vi "Dashboard Main.vi"() -> ()   [LabVIEW 2018]
uses:
  <vilib>/Utility/miscctls.llb/LVRowAndColumnTypeDef.ctl
  <vilib>/event_ctls.llb/eventvkey.ctl
  <vilib>/Rock Robotics/Network Tables/NT Read Numeric Array.vi
  <vilib>/Rock Robotics/WPI/Dashboard/WPI_DashboardLogging Global.vi
panel:
  in  "Camera Settings Right":T1={"Frame Rate"=30, "Compression"=30, "Size"=1, "DB Camera Config"=FALSE} {"Frame Rate" scale=1.0..30.0; "Compression" scale=100.0..-1.0; "Size" items=["640x480", "320x240", "160x120"]}
  in  "Camera Name Right":string(combo)="No Camera Selection"
  out "Camera Perf":string
  in  "Camera Settings":T1={"Frame Rate"=30, "Compression"=30, "Size"=1, "DB Camera Config"=FALSE} {"Frame Rate" scale=1.0..30.0; "Compression" scale=100.0..-1.0; "Size" items=["640x480", "320x240", "160x120"]}
  in  "TCP":refnum<k5>
  in  "Rec Mode":enum32{"Stop", "Record", "Playback"}(radio)
  out "Robot IP":string
  out "Image Message":string="Timeout in Camera Communications"
  in  "Dashboard Tab":T2(tab)
  in  "Select Auto":string(combo)="Select Autonomous ..."
  out "NT Connection":bool
  out "MotorChart R":cluster{"Numeric":dbl, "Numeric":dbl}(graph)
  out "MotorChart L":cluster{"Numeric":dbl, "Numeric":dbl}(graph)
  out "MotorSliders R":cluster{"MotorSlide1":dbl, "MotorSlide2":dbl} {"MotorSlide2" scale=-1.0..1.0 scale format="%#_2e"; "MotorSlide1" scale=-1.0..1.0 scale format="%#_2e"}
  out "MotorSliders L":cluster{"MotorSlide1":dbl, "MotorSlide2":dbl} {"MotorSlide2" scale=-1.0..1.0 scale format="%#_2e"; "MotorSlide1" scale=-1.0..1.0 scale format="%#_2e"}
  out "Gyro":dbl(knob) scale=0.0..360.0
  out "JS1 Z":dbl(slide) scale=-1.0..1.0 scale format="%#_2e"
  out "JS1 Graph":cluster{"X":dbl, "Y":dbl}[](graph)
  out "JS1 Buttons":T3
  out "JS2 Z":dbl(slide) scale=-1.0..1.0 scale format="%#_2e"
  out "JS2 Graph":cluster{"X":dbl, "Y":dbl}[](graph)
  out "JS2 Buttons":T3
  out "Mode":T4(ring)=enum."Auto Disabled"
  out "Right Camera Perf":cluster{"Bandwidth (Mbps)":dbl, "FPS":dbl}
  out "X Position":sgl
  out "Y Position":sgl
  out "Camera Image Right":T5(plugin-control)
  in  "DB/String 9":string
  in  "DB/String 8":string
  in  "DB/String 7":string
  in  "DB/String 6":string
  in  "DB/String 5":string
  in  "DB/String 4":string
  in  "DB/String 3":string
  in  "DB/String 2":string
  in  "DB/String 1":string
  in  "DB/String 0":string
  in  "DB/Slider 0":dbl(slide) scale=0.0..5.0
  in  "DB/Slider 1":dbl(slide) scale=0.0..5.0
  in  "DB/Slider 2":dbl(slide) scale=0.0..5.0
  in  "DB/Slider 3":dbl(slide) scale=0.0..5.0
  out "DB/LED 3":bool
  out "DB/LED 2":bool
  out "DB/LED 1":bool
  out "DB/LED 0":bool
  in  "DB/Button 3":bool
  in  "DB/Button 2":bool
  in  "DB/Button 1":bool
  in  "DB/Button 0":bool caption="New Name"
  in  "Intake Speed":dbl=0.7 min=-1.0 max=1.0 step=0.1 format="%#_2f"
  in  "Shooter Speed":dbl=0.7 min=-1.0 max=1.0 step=0.1 format="%#_2f"
  in  "Autonomous Sequence":string="Auto 1"
  in  "Select Drive Type":dbl=1.0
  in  "Drive Number":i8=2
  in  "Test Slider":dbl(slide) scale=0.0..100.0 scale format="%#_3g"
  in  "On/Off":bool caption="Solenoid"
  in  "Test Name":u16(ring) items=["Select the test to run..."]
  in  "Test Tree":string(tree)
  in  "Motor":cluster{"Value":dbl, "Enable":bool} {"Value" scale=-1.0..1.0 scale format="%#_3g"}
  out "Progress":T6 {"Test Progress" scale=0.0..100.0}
  in  "Rev/Fwd":cluster{"Forward":bool, "Reverse":bool}
  in  "Test Ring":u16(ring) items=["Monochrome", "Color"]
  out "Cmd Status":string
  in  "Execute Command":bool
  in  "Command Params":string[][](table)
  in  "Command Selection":i32(listbox)
  in  "CheckList":i32(listbox)
  out "Tree":string(tree)
  out "Camera Image":T5(plugin-control)
  out "Background":bool
  in  "Camera Name":string(combo)="No Camera Selection"
  # "HW"
  # "HW"
  # "Joysticks"
  # "Drive Motors"
  # "Front"
  # "Right"
  # "Left"
  # "Back"
  # "This tab is a great place for autonomous settings and robot-specific values.\nPlace controls and indicators inside this tab and match name to\nDashboard Variables on robot. You can also delete this comment."
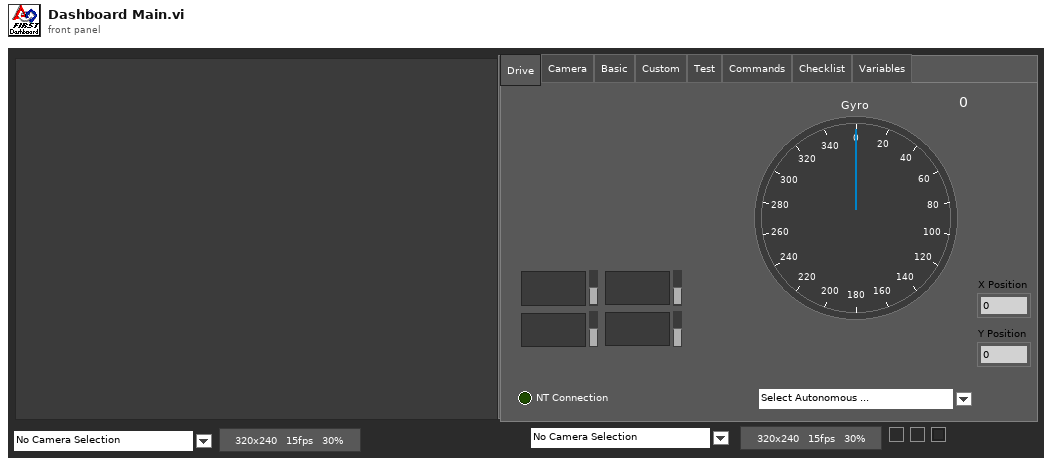
[diagram p1: front panel]
types:
  T1 = cluster{"Frame Rate":i32, "Compression":i32, "Size":u16, "DB Camera Config":bool}
  T2 = enum32{"Drive", "Camera", "Basic", "Custom", "Test", "Commands", "Checklist", "Variables"}
  T3 = cluster{bool, bool, bool, bool, bool, bool, bool, bool, bool, bool, bool, bool}
  T4 = enum8{"Tele-Op Disabled", "Tele-Op Enabled", "Auto Disabled", "Auto Enabled", "Test Disabled", "Test Enabled", "Disconnected", "No Code", "E-Stop"}
  T5 = typedef "IMAQ Image.ctl" = refnum<image>
  T6 = cluster{"Test Progress":u8, "Test Progress Text":string}
  T7 = cluster{"Save Path":path, "Interval (s)":dbl, "Keep":i32}
  T8 = typedef "Image Type" = u32
  T9 = cluster{"IDs":cluster{"RPC field ID":u16, "Unique ID":u16}, "String":string}
  T10 = cluster{"Camera Image":refnum<vi>, "Dashboard Tab":refnum<vi>, "Background":refnum<vi>, "Rec Mode":refnum<vi>, "Test Slider":refnum<vi>, "On/Off ":refnum<vi>, "Test Ring":refnum<vi>, "Rev/Fwd":refnum<vi>, "Test Name":refnum<vi>, "Motor":refnum<vi>, "Progress":refnum<vi>, "CheckList":refnum<vi>, "Tree":refnum<vi>, "Test Tree":refnum<vi>, "Command Params":refnum<vi>, "Command Selection":refnum<vi>, "Execute Command":refnum<vi>, "Cmd Status":refnum<vi>, "Camera Settings":refnum<vi>, "Camera Name":refnum<vi>, "Camera Perf":refnum<vi>, "Camera Settings Right":refnum<vi>, "Camera Name Right":refnum<vi>, "Camera Image Right":refnum<vi>}
  T11 = cluster{"Global Rectangle":i32[], "Contours":cluster{"Contour Type":u32, "ROI Type":u32, "Points":i32[]}[]}
  T12 = cluster{"Camera Name Right":string, string, "Saved DB Images Info":cluster{"Save Path":path, "Interval (s)":dbl, "Keep":i32}}
  T13 = cluster{"Error Strings":string, "Disable Counts":cluster{u16, u16}, "Rail Faults":cluster{u16, u16, u16}, "Robot IP":string, "DB Mode":u8, "Event Info":cluster{"Name":string, "Type":u8, "Number":u16, "Replay":u8}}
  T14 = cluster{"Storage":cluster{"Disk Free":u64, "RAM Block":u32, "RAM free":u32}, "CPU Utilization":cluster{"CPU % ISR":sgl, "CPU % Time Crit":sgl, "CPU % Timed Str":sgl, "CPU % High":sgl, "CPU % Above":sgl, "CPU % Normal":sgl, "CPU % Low":sgl}, "CAN":cluster{"% Bus Utilization":sgl, "Bus Off Cnt":u32, "TX_FIFO Full Cnt":u32, "Receive Error Cnt":u8, "Transmit Error Cnt":u8}, "HID":cluster{"HID Outputs":u32, "Rumble Low":u16, "Rumble High":u16}[]}
  T15 = cluster{"Status bits":cluster{"Test Mode":bool, "Autonomous":bool, "Enabled":bool, "Code Start":bool, "Brownout":bool, "Reserved 2":bool, "Reserved 3":bool, "E-Stop":bool}, "Code Trace":cluster{"Disabled":bool, "TeleOp":bool, "Auto":bool, "Test":bool}, "Controller Type":enum16{"unknown", "cRIO", "roboRio"}, "Code?":enum16{"unknown", "noCode", "code"}, "Battery V":dbl}
  T16 = cluster{"Control Bits":cluster{"TestMode":bool, "Autonomous":bool, "Enabled":bool, "FMS Present":bool, bool, bool, bool, "E-Stop":bool}, "Team Station ":u8, "Countdown":sgl, "Joystick Values":cluster{"Axes":dbl[], "Buttons":bool[], "POVs":i16[]}[]}
  T17 = cluster{"Axes":dbl[], "Buttons":bool[], "POVs":i16[]}[]
  T18 = cluster{"Axes":dbl[], "Buttons":bool[], "POVs":i16[]}
  T19 = cluster{"Buttons[0]":bool, "Buttons[1]":bool, "Buttons[2]":bool, "Buttons[3]":bool, "Buttons[4]":bool, "Buttons[5]":bool, "Buttons[6]":bool, "Buttons[7]":bool, "Buttons[8]":bool, "Buttons[9]":bool, "Buttons[10]":bool, "Buttons[11]":bool}
  T20 = cluster{"Camera Name":string, string, "Saved DB Images Info":cluster{"Save Path":path, "Interval (s)":dbl, "Keep":i32}}
  T21 = cluster{"Position":cluster{"x":sgl, "y":sgl}, "Angle":sgl, "Scale":sgl, "Score":sgl, "Bounding Box":cluster{"x":sgl, "y":sgl}[]}[]
  T22 = cluster{"Position":cluster{"x":sgl, "y":sgl}, "Angle":sgl, "Scale":sgl, "Score":sgl, "Bounding Box":cluster{"x":sgl, "y":sgl}[]}
  T23 = cluster{"Operation":enum16{"Update", "Clear"}, "Color Box":u32}[]
  T24 = typedef "eventvkey.ctl" = enum16{"ASCII", "Enter", "Return", "Shift", "Ctrl", "Alt", "Cmd", "Opt", "Caps", "NumLock", "Clear", "Break", "Up", "Down", "Left", "Right", "Insert", "Delete", "Home", "End", "PageUp", "PageDown", "Escape", "Help", "Pause", "ScrollLock", "F1", "F2", "F3", "F4", "F5", "F6", "F7", "F8", "F9", "F10", "F11", "F12", "F13", "F14", "F15", "F16", "F17", "F18", "F19", "F20", "F21", "F22", "F23", "F24", "Play", "VolumeUp", "VolumeDown", "Mute", "Two Byte Char"}
  T25 = cluster{"Image Size":bool, "Image Type":bool, "Pixel Value":bool, "ROI Information":bool, "Zoom Factor":bool}
  T26 = cluster{"Operation":enum16{"Update", "Clear"}, "Color Box":u32}
  T27 = typedef "LVRowAndColumnTypeDef.ctl" = cluster{"Row":i32, "Column":i32}
  T28 = cluster{"Shift":bool, "Ctrl":bool, "Alt":bool, "Cmd":bool, "Opt":bool}
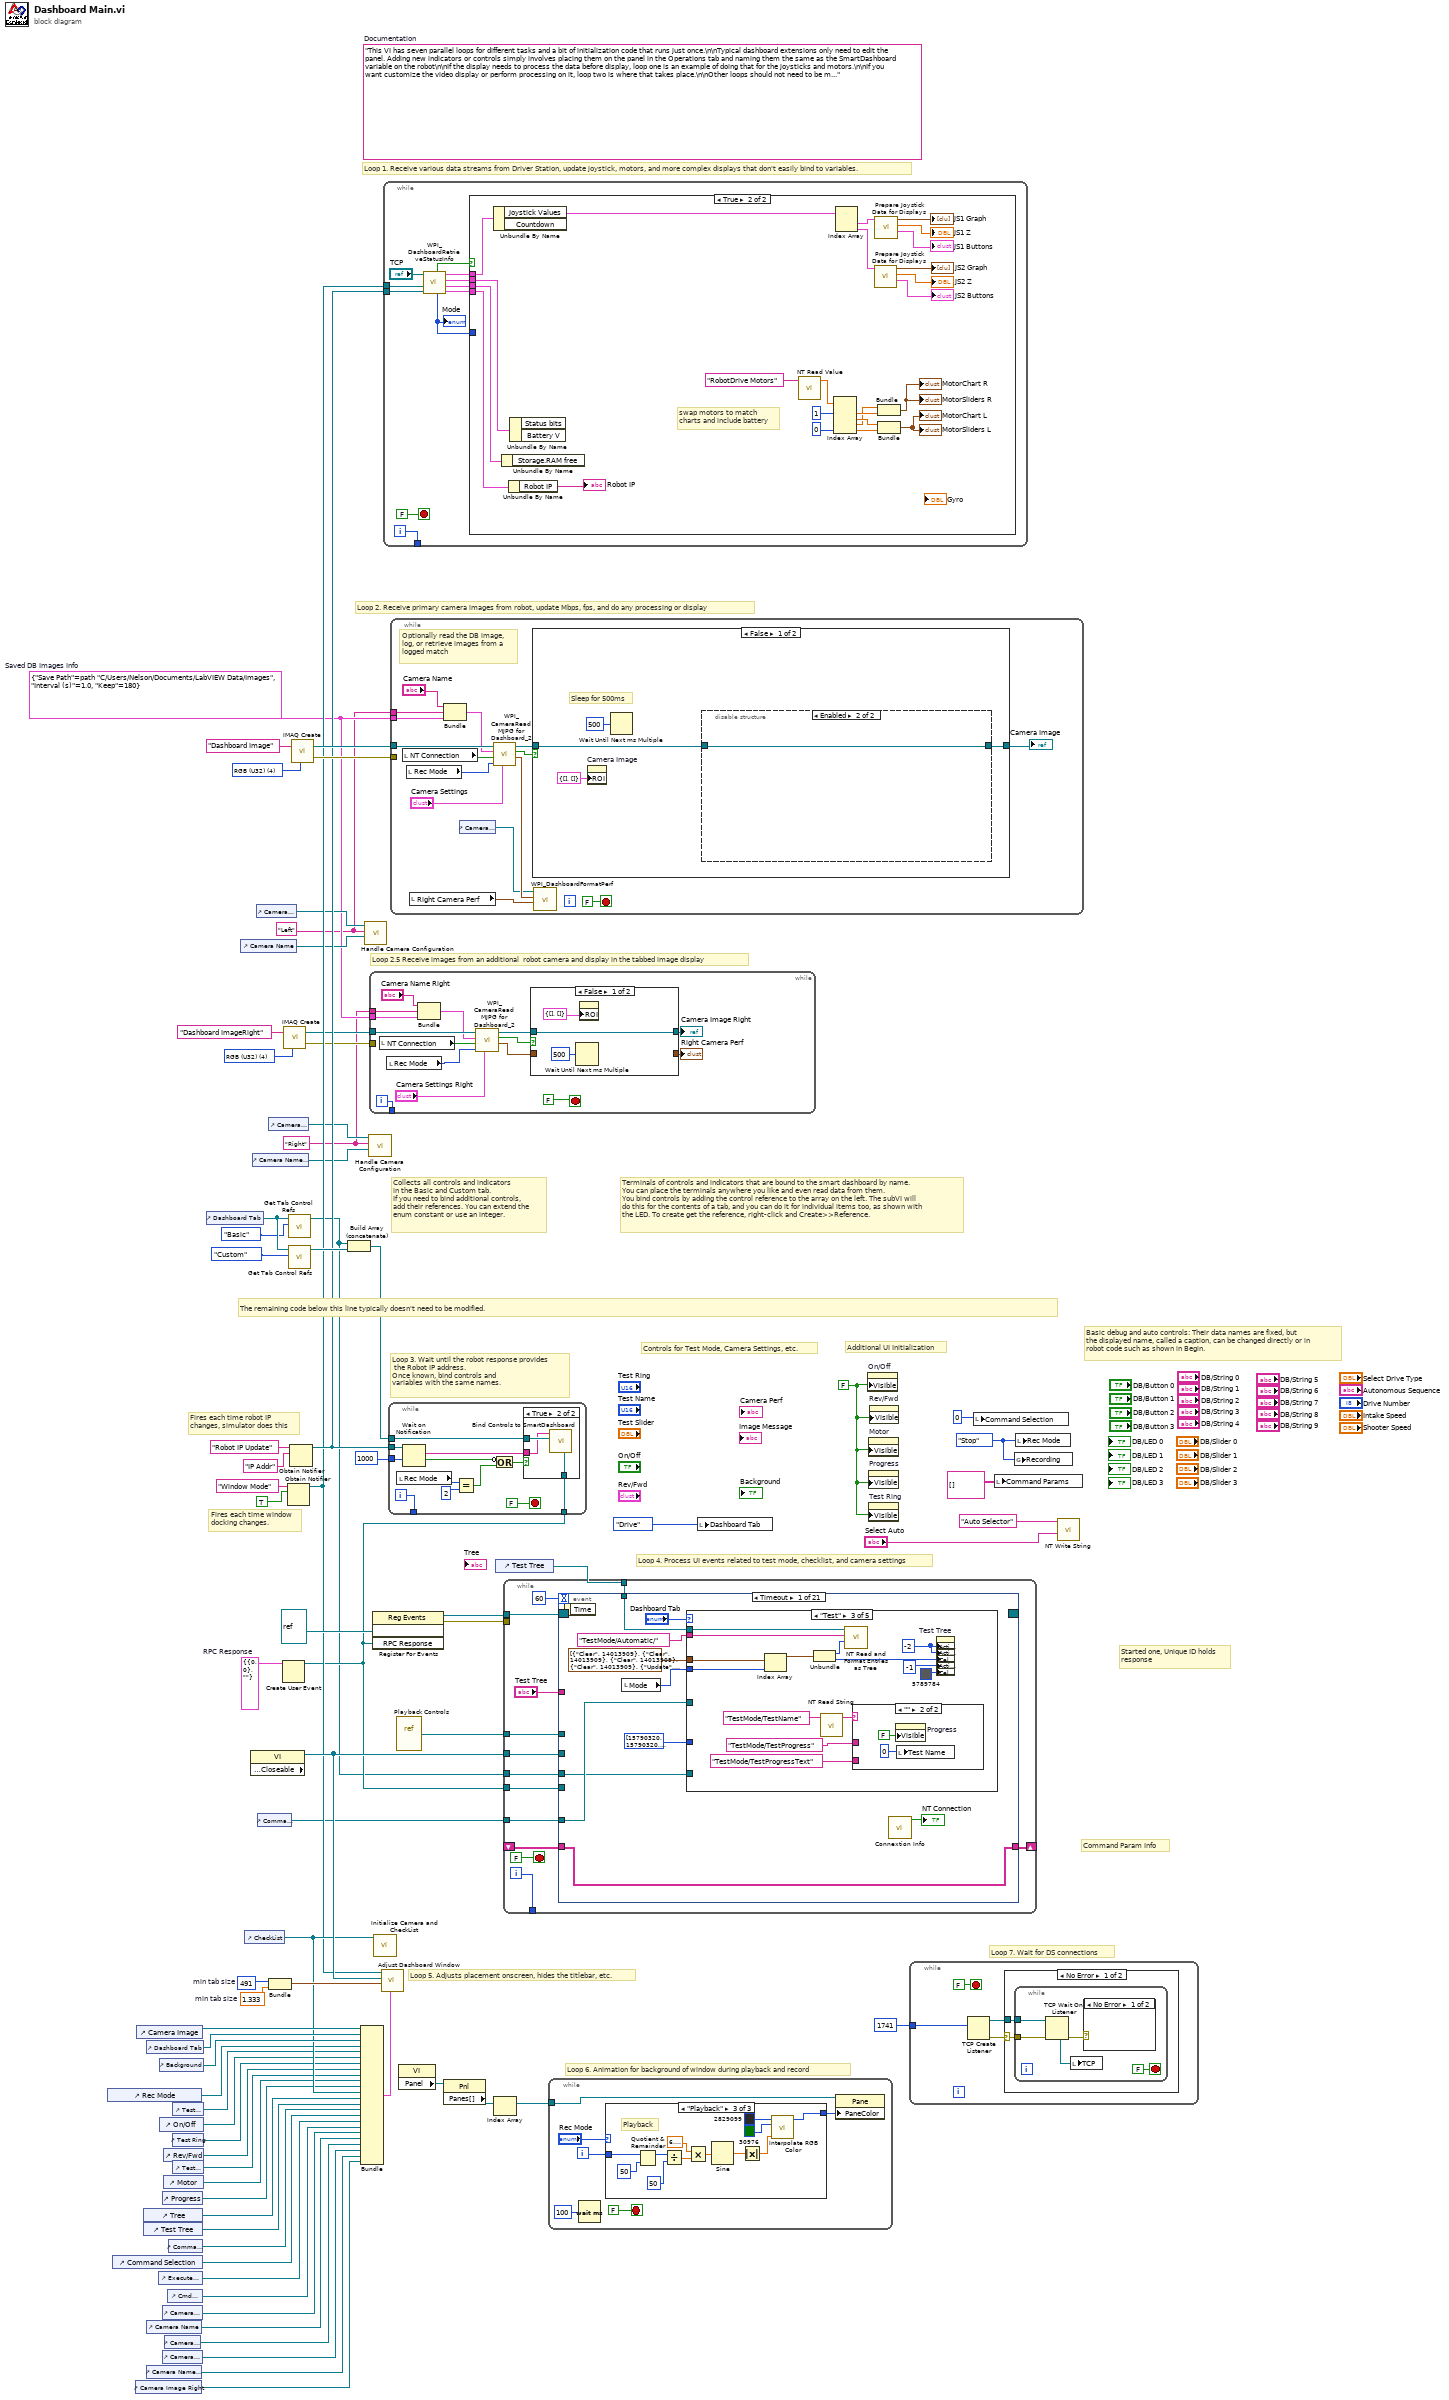
[diagram p0: block diagram]
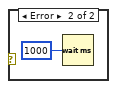
[diagram p3: hidden frame]
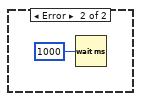
[diagram p4: hidden frame]
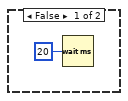
[diagram p5: hidden frame]
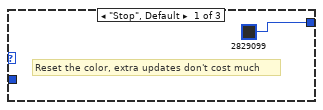
[diagram p6: hidden frame]
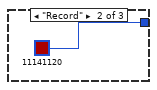
[diagram p7: hidden frame]
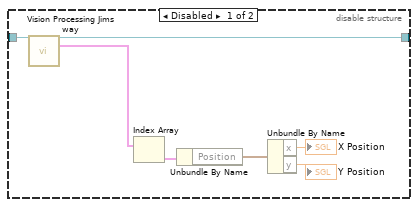
[diagram p9: hidden frame]
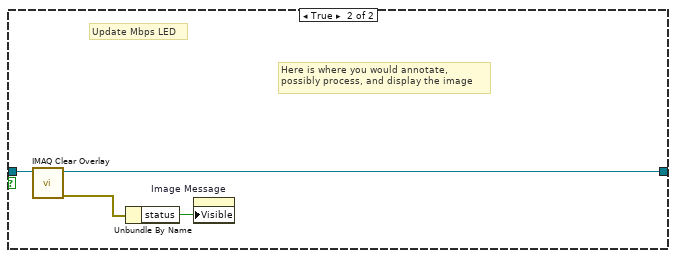
[diagram p10: hidden frame]
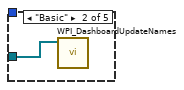
[diagram p12: hidden frame]
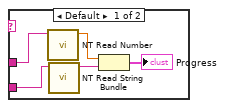
[diagram p13: hidden frame]
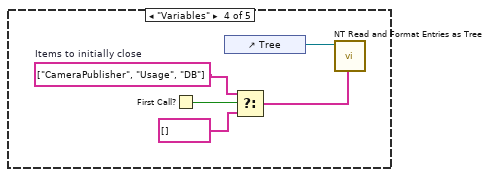
[diagram p14: hidden frame]
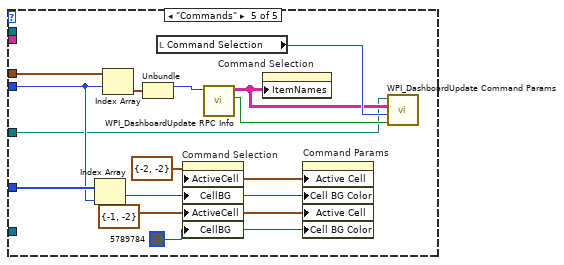
[diagram p15: hidden frame]
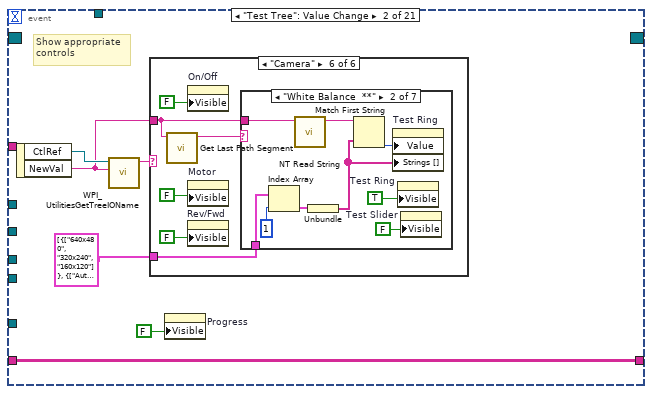
[diagram p16: hidden frame]
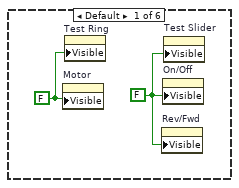
[diagram p17: hidden frame]
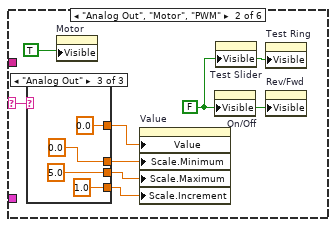
[diagram p18: hidden frame]
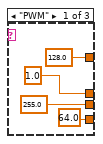
[diagram p19: hidden frame]
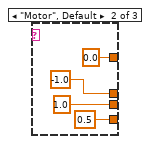
[diagram p20: hidden frame]
diagram:
  w3 = T7 {"Save Path"=path "C:/Users/Nelson/Documents/LabVIEW Data/Images", "Interval (s)"=1.0, "Keep"=180}  # Saved DB Images Info
  w2 = "Right"
  w1 = "Left"
  w13 = T8 4 items=["Grayscale (U8)", "Grayscale (I16)", "Grayscale (SGL)", "Complex (CSG)", "RGB (U32)", "HSL (U32)", "RGB (U64)"] ("Image Type")
  w29 = T9 {"IDs"={"RPC field ID"=0, "Unique ID"=0}, "String"=""}  # RPC Response
  w52 = 491  # min tab size
  w51 = 1.333  # min tab size
  w59 = enum32{"Stop", "Record", "Playback"}."Stop" ("Rec Mode")
  w36 = FALSE ("Visible")
  (unwired) "This VI has seven parallel loops for different tasks and a bit of initialization code that runs just once.\n\nTypical dashboard extensions only need to edit the panel. Adding new indicators or controls simply involves placing them on the panel in the Operations tab and naming them the same as the SmartDashboard variable on the robot\n\nIf the display needs to process the data before display, loop one is an example of doing that for the joysticks and motors.\n\nIf you want customize the video display or perform processing on it, loop two is where that takes place.\n\nOther loops should not need to be modified. They are pretty standard, and document the task they perform."  # Documentation
  w76 = T8 4 items=["Grayscale (U8)", "Grayscale (I16)", "Grayscale (SGL)", "Complex (CSG)", "RGB (U32)", "HSL (U32)", "RGB (U64)"] ("Image Type")
  # "Loop 2.5 Receive images from an additional  robot camera and display in the tabbed image display"
  # "Command Param Info"
  # "Started one, Unique ID holds\nresponse"
  # "Loop 7. Wait for DS connections"
  # "Basic debug and auto controls: Their data names are fixed, but\nthe displayed name, called a caption, can be changed directly or in\nrobot code such as shown in Begin."
  # "Controls for Test Mode, Camera Settings, etc."
  # "Additional UI Initialization"
  # "Loop 6. Animation for background of window during playback and record"
  # "Fires each time robot IP\nchanges, simulator does this"
  # "Fires each time window\ndocking changes."
  # "Collects all controls and indicators\nin the Basic and Custom tab.\nIf you need to bind additional controls,\nadd their references. You can extend the\nenum constant or use an integer."
  # "The remaining code below this line typically doesn't need to be modified."
  # "Loop 4. Process UI events related to test mode, checklist, and camera settings"
  # "Terminals of controls and indicators that are bound to the smart dashboard by name.\nYou can place the terminals anywhere you like and even read data from them.\nYou bind controls by adding the control reference to the array on the left. The subVI will\ndo this for the contents of a tab, and you can do it for individual items too, as shown with\nthe LED. To create get the reference, right-click and Create>>Reference."
  # "Loop 3. Wait until the robot response provides\n the Robot IP address.\nOnce known, bind controls and\nvariables with the same names."
  # "Loop 5. Adjusts placement onscreen, hides the titlebar, etc."
  # "Loop 1. Receive various data streams from Driver Station, update joystick, motors, and more complex displays that don't easily bind to variables."
  # "Loop 2. Receive primary camera images from robot, update Mbps, fps, and do any processing or display"
  n1 = control-ref of="Rec Mode"() -> (w42:refnum<vi>)
  n2 = control-ref of="Command Selection"() -> (w28:refnum<vi>)
  n3 = control-ref of="Camera Image Right"() -> (w6:refnum<vi>)
  n4 = control-ref of="Camera Image"() -> (w54:refnum<vi>)
  n5 = control-ref of="Tree"() -> (w46:refnum<vi>)
  n6 = control-ref of="Test Tree"() -> (w45:refnum<vi>)
  n7 = control-ref of="Dashboard Tab"() -> (w53:refnum<vi>)
  n8 = control-ref of="Camera Name"() -> (w19:refnum<vi>)
  n9 = control-ref of="Camera Name Right"() -> (w7:refnum<vi>)
  n10 = control-ref of="Execute Command"() -> (w30:refnum<vi>)
  n11 = control-ref of="Background"() -> (w49:refnum<vi>)
  n12 = control-ref of="On/Off"() -> (w40:refnum<vi>)
  n13 = control-ref of="Progress"() -> (w37:refnum<vi>)
  n14 = control-ref of="Camera Settings"() -> (w20:refnum<vi>)
  n15 = control-ref of="Camera Settings Right"() -> (w8:refnum<vi>)
  n16 = control-ref of="Rev/Fwd"() -> (w38:refnum<vi>)
  n17 = control-ref of="Motor"() -> (w43:refnum<vi>)
  n18 = control-ref of="Camera Perf"() -> (w18:refnum<vi>)
  n19 = control-ref of="Cmd Status"() -> (w24:refnum<vi>)
  n20 = control-ref of="Command Params"() -> (w31:refnum<vi>)
  n21 = control-ref of="Test Slider"() -> (w41:refnum<vi>)
  n22 = control-ref of="Test Ring"() -> (w39:refnum<vi>)
  n23 = control-ref of="Test Name"() -> (w44:refnum<vi>)
  n24 = control-ref of="Dashboard Tab"() -> (w57:refnum<vi>)
  n25 = control-ref of="Camera Name"() -> (w21:refnum<vi>)
  n26 = control-ref of="CheckList"() -> (w47:refnum<vi>)
  n27 = property class="VI" props=["Front Panel.Closeable"]() -> (reference out=w58:refnum<vi>)  [unwired: 2 in, 2 out]
  n28 = control-ref of="Camera Name Right"() -> (w9:refnum<vi>)
  n29 = control-ref of="Camera Settings"() -> (w22:refnum<vi>)
  n30 = control-ref of="Command Params"() -> (w23:refnum<vi>)
  n31 = control-ref of="Camera Settings Right"() -> (w10:refnum<vi>)
  n32 = Bundle("min tab size"=w52, "min tab size"=w51) -> (w50:cluster{"min tab size":i32, "min tab size":dbl})  [unwired: 1 in]
  n33 = Create User Event(user event datatype=w29) -> (user event=w25:refnum<user-event>)  [unwired: 1 in, 1 out]
  n34 = call "IMAQ Create"("Image Name"="Dashboard ImageRight", "Image Type"=w13) -> ("New Image"=w12:T5, "error out"=w11:errorcluster)  [unwired: 2 in, 1 out]
  n35 = Obtain Notifier(name (unnamed)="Window Mode", notification data type=TRUE) -> (notifier out=w34:refnum<notifier>)  [unwired: 2 in, 2 out]
  n36 = call <vilib>:"Get Tab Control Refs.vi"("Page Index"=T2."Basic" ("Dashboard Tab"), "TabControl in"=w57) -> ("ControlsOnPage"=w17:refnum<vi>[])  [unwired: 9 in]
  n37 = call <vilib>:"Get Tab Control Refs.vi"("Page Index"=T2."Custom" ("Dashboard Tab"), "TabControl in"=w57) -> ("ControlsOnPage"=w56:refnum<vi>[])  [unwired: 9 in]
  n38 = Obtain Notifier(name (unnamed)="Robot IP Update", notification data type="IP Addr" ("name (unnamed)")) -> (notifier out=w35:refnum<notifier>)  [unwired: 2 in, 2 out]
  n39 = call "IMAQ Create"("Image Name"="Dashboard Image", "Image Type"=w76) -> ("New Image"=w74:T5, "error out"=w73:errorcluster)  [unwired: 2 in, 1 out]
  n40 = Build Array (concatenate)(w17, w56) -> (w55:refnum<vi>[])
  n41 = Bundle("Camera Image"=w54, "Dashboard Tab"=w53, "Background"=w49, "Rec Mode"=w42, "Test Slider"=w41, "On/Off"=w40, "Test Ring"=w39, "Rev/Fwd"=w38, "Test Name"=w44, "Motor"=w43, "Progress"=w37, "CheckList"=w47, "Tree"=w46, "Test Tree"=w45, "Command Params"=w31, "Command Selection"=w28, "Execute Command"=w30, "Cmd Status"=w24, "Camera Settings"=w20, "Camera Name"=w19, "Camera Perf"=w18, "Camera Settings Right"=w8, "Camera Name Right"=w7, "Camera Image Right"=w6) -> (w48:T10)  [unwired: 1 in]
  n42 = call "Handle Camera Configuration.vi"("CameraNameRef"=w21, "Display Name"=w1, "ClusterRef"=w22) -> ()  [unwired: 9 in]
  n43 = call "Handle Camera Configuration.vi"("CameraNameRef"=w9, "Display Name"=w2, "ClusterRef"=w10) -> ()  [unwired: 9 in]
  n44 = while {
    tunnel: w12 -> [w91]
    tunnel: w11 -> [_]
    tunnel: [w86] -> _
    tunnel: w3 -> [w82]
    tunnel: w2 -> [w79]
    i -> [w86]
    stop <- FALSE stop-if-true
    n45 = local read "NT Connection"() -> (w83:bool)
    n46 = local read "Rec Mode"() -> (w90:enum32{"Stop", "Record", "Playback"})
    n47 = Bundle("Camera Name Right"="Camera Name Right", w79, "Saved DB Images Info"=w82) -> (w81:T12)  [unwired: 1 in]
    n48 = call <vilib>:"WPI_CameraRead MJPG for Dashboard_2.vi"("Camera Settings"="Camera Settings Right", "Rec Mode"=w90, "NT Connection"=w83, "Capture Info"=w81, "Image in"=w91) -> ("perf info"=w77:cluster{"Bandwidth (Mbps)":dbl, "fps":dbl}, "Active"=w85:bool, "Image\\ out"=w88:T5)  [unwired: 4 in]
    n49 = case shown="False" w85 {
      tunnel: w88 -> [w93 w96]
      tunnel: [w93 w96] -> w84
      tunnel: [_ w95] -> w78
      tunnel: w77 -> [_ w95]
      frame False {
        n50 = Wait Until Next ms Multiple(millisecond multiple=u32 500) -> ()  [unwired: 1 out]
        n51 = property on="Camera Image Right" class="ImageControl"("ROI"=T11 {"Global Rectangle"=[], "Contours"=[]}) -> ()  [unwired: 2 in, 2 out]
      }
      frame True {
      }
    }
    "Camera Image Right" <- w84
    "Right Camera Perf" <- w78
  }
  n52 = register-events(refnum<vi> refnum, w25) -> (reference out=w63:refnum<event-registration>, error out=w62:errorcluster)  [unwired: 2 in]
  n53 = call "Initialize Camera and CheckList.vi"("ListBox in"=w47) -> ()  [unwired: 11 in]
  n54 = call "Adjust Dashboard Window.vi"("Sizing Refnums"=w48, "Size Constraints"=w50, "VI"=w58, "WIn Mode"=w34) -> ()  [unwired: 8 in]
  n55 = while {
    tunnel: [w106] -> _
    tunnel: w35 -> [w100]
    tunnel: w34 -> [w97]
    i -> [w106]
    stop <- FALSE stop-if-true
    n56 = call <vilib>:"WPI_DashboardRetrieveStatusInfo.vi"("Binding Refnum"=w100, "Window Mode Notifier"=w97, "TCP Cnx"="TCP") -> ("Power and Errors"=w101:T13, "Robot Metrics"=w104:T14, "Status Info"=w105:T15, "Control Info"=w102:T16, "Robot Mode"=w99:T4, "Process?"=w103:bool)  [unwired: 3 in]
    "Mode" <- w99
    n57 = case shown="True" w103 {
      tunnel: w105 -> [_ w132]
      tunnel: w104 -> [_ w131]
      tunnel: w102 -> [_ w130]
      tunnel: w101 -> [_ w129]
      tunnel: w99 -> [_ _]
      frame False {
        n58 = Wait (ms)(milliseconds to wait=u32 20) -> ()  [unwired: 1 out]
      }
      frame True {
        # "swap motors to match\ncharts and include battery"
        n59 = Unbundle By Name(w130) -> ("Joystick Values"=w120:T17)  [unwired: 1 out]
        n60 = Unbundle By Name(w131) -> ()  [unwired: 1 out]
        n61 = Unbundle By Name(w129) -> ("Robot IP"=→"Robot IP":string)
        n62 = Unbundle By Name(w132) -> ()  [unwired: 2 out]
        n63 = call-poly <vilib>:"NT Read Value.vi"("Name"="RobotDrive Motors") -> ("Numeric Array"=w110:dbl[])  [unwired: 9 in, 1 out]
        n64 = Index Array(array=w110, index #1=1, index #4=0) -> (element #1=w124:dbl, element #2=w125:dbl, element #3=w123:dbl, element #4=w128:dbl)  [unwired: 2 in]
        n65 = Index Array(array=w120) -> (element #1=w119:T18, element #2=w115:T18)  [unwired: 2 in]
        n66 = call "Prepare Joystick Data for Displays.vi"("Joystick Values"=w115) -> ("Buttons"=→"JS2 Buttons":T19, "Z Axis"=→"JS2 Z":dbl, "Cartesian Data"=→"JS2 Graph":cluster{"X axis":dbl, "X axis":dbl}[])  [unwired: 8 in]
        n67 = call "Prepare Joystick Data for Displays.vi"("Joystick Values"=w119) -> ("Buttons"=→"JS1 Buttons":T19, "Z Axis"=→"JS1 Z":dbl, "Cartesian Data"=→"JS1 Graph":cluster{"X axis":dbl, "X axis":dbl}[])  [unwired: 8 in]
        n68 = Bundle("Numeric"=w123, "Numeric"=w124) -> (→"MotorChart R" →"MotorSliders R":cluster{"Numeric":dbl, "Numeric":dbl})  [unwired: 1 in]
        n69 = Bundle("Numeric"=w125, "Numeric"=w128) -> (→"MotorChart L" →"MotorSliders L":cluster{"Numeric":dbl, "Numeric":dbl})  [unwired: 1 in]
      }
    }
  }
  n70 = while {
    tunnel: w55 -> [w144]
    tunnel: w35 -> [w142]
    tunnel: [w140] -> _
    tunnel: u32 1000 ("milliseconds to wait") -> [w139]
    tunnel: w25 -> [w133]
    i -> [w140]
    stop <- FALSE stop-if-true
    n71 = local read "Rec Mode"() -> (w135:enum32{"Stop", "Record", "Playback"})
    n72 = Wait on Notification(notifier=w142, timeout in ms (-1)=w139) -> (notification=w141:string, timed out?=w137:bool)  [unwired: 2 in, 2 out]
    n73 = Equal?(x=w135, y=u16 2 ("Rec Mode")) -> (x = y?=w136:bool)
    n74 = Compound Arithmetic op=OR(invert w137, w136) -> (w138:bool)
    n75 = case shown="True" w138 {
      tunnel: w144 -> [_ w147]
      tunnel: w141 -> [_ w146]
      tunnel: w133 -> [_ w145]
      frame False {
      }
      frame True {
        n76 = call <vilib>:"Bind Controls to SmartDashboard.vi"("RPC ref"=w145, "Bound Control Refs"=w147, "Server IP Address"=w146) -> ()  [unwired: 9 in]
      }
    }
  }
  n77 = while {
    tunnel: w74 -> [w161]
    tunnel: w73 -> [_]
    tunnel: w3 -> [w154]
    tunnel: w1 -> [w151]
    stop <- FALSE stop-if-true
    # "Optionally read the DB image,\nlog, or retrieve images from a\nlogged match"
    n78 = local read "NT Connection"() -> (w155:bool)
    n79 = local read "Rec Mode"() -> (w158:enum32{"Stop", "Record", "Playback"})
    n80 = local read "Right Camera Perf"() -> (w149:cluster{"Bandwidth (Mbps)":dbl, "FPS":dbl})
    n81 = Bundle("Camera Name"="Camera Name", w151, "Saved DB Images Info"=w154) -> (w153:T20)  [unwired: 1 in]
    n82 = control-ref of="Camera Perf"() -> (w148:refnum<vi>)
    n83 = call <vilib>:"WPI_CameraRead MJPG for Dashboard_2.vi"("Camera Settings"="Camera Settings", "Rec Mode"=w158, "NT Connection"=w155, "Capture Info"=w153, "Image in"=w161) -> ("perf info"=w150:cluster{"Bandwidth (Mbps)":dbl, "fps":dbl}, "Active"=w159:bool, "Image\\ out"=w160:T5)  [unwired: 4 in]
    n84 = case shown="False" w159 {
      tunnel: w160 -> [w164 w176]
      tunnel: [w163 w175] -> w156
      frame False {
        # "Sleep for 500ms"
        n85 = property on="Camera Image" class="ImageControl"("ROI"=T11 {"Global Rectangle"=[], "Contours"=[]}) -> ()  [unwired: 2 in, 2 out]
        n86 = Wait Until Next ms Multiple(millisecond multiple=u32 500) -> ()  [unwired: 1 out]
        n87 = disable-structure shown="Enabled" {
          disable-tunnel: w164 -> [w169 w174]
          disable-tunnel: [w168 w174] -> w163
          frame Disabled {
            n88 = call "Vision Processing Jims way.vi"("Image In"=w169) -> ("Image Out"=w168:T5, "Calibrated Matches (Pattern Matching 1)"=w167:T21)  [unwired: 22 in, 3 out]
            n89 = Index Array(array=w167) -> (element=w173:T22)  [unwired: 1 in]
            n90 = Unbundle By Name(w173) -> ("Position"=w172:cluster{"x":sgl, "y":sgl})
            n91 = Unbundle By Name(w172) -> ("x"=→"X Position":sgl, "y"=→"Y Position":sgl)
          }
          frame Enabled {
          }
        }
      }
      frame True {
        # "Here is where you would annotate,\npossibly process, and display the image"
        # "Update Mbps LED"
        n92 = call "IMAQ Clear Overlay"("Image"=w176) -> ("error out"=w177:errorcluster, "Image Out"=w175:T5)  [unwired: 2 in, 7 out]
        n93 = Unbundle By Name(w177) -> ("status"=w178:bool)
        n94 = property on="Image Message" class="Str"("Visible"=w178) -> ()  [unwired: 2 in, 2 out]
      }
    }
    "Camera Image" <- w156
    n95 = call <vilib>:"WPI_DashboardFormatPerf.vi"("Right Camera Perf"=w149, "Performance"=w150, "String in"=w148) -> ()  [unwired: 9 in]
  }
  n96 = vi-ref "Playback Controls.vi"() -> (w64:refnum<vi>)
  n97 = property class="VI"() -> ("Panel"=w66:refnum<vi>)  [unwired: 2 in, 2 out]
  n98 = property class="Pnl"(reference=w66) -> ("Panes[]"=w67:refnum<vi>[])  [unwired: 1 in, 2 out]
  n99 = Index Array(array=w67) -> (element=w65:refnum<vi>)  [unwired: 1 in]
  n100 = control-ref of="Test Tree"() -> (w68:refnum<vi>)
  n101 = while {
    tunnel: [w188] -> _
    tunnel: w68 -> [w187]
    tunnel: w64 -> [w186]
    tunnel: w63 -> [w185]
    tunnel: w62 -> [_]
    tunnel: w58 -> [w184]
    tunnel: w25 -> [w183]
    tunnel: w23 -> [w182]
    shift-right: [w181] -> _
    shift-left: _ -> [w180]
    tunnel: w17 -> [w179]
    i -> [w188]
    stop <- FALSE stop-if-true
    n102 = event shown="[0] Timeout" {
      selector: w185 -> [_ _ _ _ _ _ _ _ _ _ _ _ _ _ _ _ _ _ _ _ _]
      dyn-events: [_ _ _ _ _ _ _ _ _ _ _ _ _ _ _ _ w448 _ _ _ _] -> _
      timeout: u32 60 ("milliseconds to wait") -> [_ _ _ _ _ _ _ _ _ _ _ _ _ _ _ _ _ _ _ _ _]
      tunnel: w187 -> [w200 _ _ _ _ _ _ _ _ _ _ _ _ _ _ _ _ _ _ _ _]
      tunnel: "Test Tree" -> [_ _ _ _ _ _ _ _ _ _ _ w415 w423 w425 w429 w437 _ _ _ _ _]
      tunnel: w186 -> [_ _ _ _ _ _ _ _ _ _ _ _ _ _ _ _ w450 _ w468 _ _]
      tunnel: w184 -> [_ _ _ _ _ _ _ _ _ _ _ _ _ _ _ _ w446 _ _ _ _]
      tunnel: w183 -> [_ _ _ _ _ _ _ _ _ _ _ _ _ _ _ _ w444 _ _ _ _]
      tunnel: w182 -> [w195 _ _ _ _ _ w366 _ _ _ _ _ _ _ _ _ _ _ _ _ _]
      tunnel: [w194 w243 w345 w350 w359 w363 w364 w373 w383 w390 w402 w414 w421 w424 w428 w436 w443 w463 w465 w469 w482] -> w181
      tunnel: w180 -> [w194 w243 w345 w350 w359 w363 w364 _ _ w390 w402 w414 w421 w424 w428 w436 w443 w463 w465 w469 w482]
      tunnel: w179 -> [w192 _ _ _ _ _ _ _ _ _ _ _ _ _ _ _ _ _ _ _ _]
      event Timeout {
        n103 = event-data() -> ()  [unwired: 1 in, 1 out]
        n104 = local read "Mode"() -> (w197:T4)
        n105 = case shown="\"Test\"" "Dashboard Tab" {
          tunnel: w200 -> [_ _ w216 _ _]
          tunnel: "TestMode/Automatic/" ("Name Pattern") -> [_ _ w215 _ _]
          tunnel: T23 [{"Operation"=enum."Clear", "Color Box"=14013909}, {"Operation"=enum."Clear", "Color Box"=14013909}, {"Operation"=enum."Clear", "Color Box"=14013909}, {"Operation"=enum."Clear", "Color Box"=14013909}, {"Operation"=enum."Update", "Color Box"=14013909}, {"Operation"=enum."Update", "Color Box"=16777215}, {"Operation"=enum."Clear", "Color Box"=14013909}, {"Operation"=enum."Clear", "Color Box"=14013909}, {"Operation"=enum."Clear", "Color Box"=14013909}] -> [_ _ w208 _ w236]
          tunnel: w197 -> [_ _ w207 _ w235]
          tunnel: u32[] [15790320, 15790320, 15790320, 15790320, 16777215, 16777215, 15790320, 15790320, 15790320] -> [_ _ _ _ w241]
          tunnel: w195 -> [_ _ _ _ w229]
          tunnel: w192 -> [_ w202 _ _ _]
          frame "Custom", Default {
          }
          frame "Basic" {
            n106 = call <vilib>:"WPI_DashboardUpdateNames.vi"("Controls on Tab"=w202) -> ()  [unwired: 11 in]
          }
          frame "Test" {
            w214 = -2 ("Active Item:Row Number")
            n107 = Index Array(array=w208, index=w207) -> (element=w209:T26)
            n108 = Unbundle(w209) -> ("Operation"=w210:enum16{"Update", "Clear"}, "Color Box"=w211:u32)
            n109 = call <vilib>:"NT Read String.vi"("Name"="TestMode/TestName") -> ("String"=w205:string)  [unwired: 9 in, 1 out]
            n110 = call <vilib>:"NT Read and Format Entries as Tree.vi"("Operation"=w210, "Name Pattern"=w215, "Tree Refnum"=w216) -> ()  [unwired: 7 in, 2 out]
            n111 = case shown="\"\"" w205 {
              tunnel: "TestMode/TestProgress" ("Name") -> [w218 _]
              tunnel: "TestMode/TestProgressText" ("Name") -> [w217 _]
              frame Default {
                n112 = call <vilib>:"NT Read Number.vi"("Name"=w218) -> ("Numeric"=w219:dbl)  [unwired: 9 in, 1 out]
                n113 = call <vilib>:"NT Read String.vi"("Name"=w217) -> ("String"=w220:string)  [unwired: 9 in, 1 out]
                n114 = Bundle("Numeric"=w219, "String"=w220) -> (→"Progress":cluster{"Numeric":dbl, "String":string})  [unwired: 1 in]
              }
              frame "" {
                n115 = property on="Progress" class="Clust (strict)"("Visible"=FALSE) -> ()  [unwired: 2 in, 2 out]
                n116 = local write "Test Name"(u16 0) -> ()
              }
            }
            n117 = property on="Test Tree" class="Tree (strict)"("Active Item Row Number"=w214, "ActiveColNum"=w214, "CellBG"=w211, "Active Item Row Number"=-1 ("Active Item:Row Number"), "CellBG"=u32 5789784 ("Color Box")) -> ()  [unwired: 2 in, 2 out]
          }
          frame "Variables" {
            w226 = string[] ["CameraPublisher", "Usage", "DB"]  # Items to initially close
            n118 = First Call?() -> (First Call?: T/F=w227:bool)
            n119 = control-ref of="Tree"() -> (w228:refnum<vi>)
            n120 = Select(t=w226, s=w227, f=string[] []) -> (s? t:f=w224:string[])
            n121 = call <vilib>:"NT Read and Format Entries as Tree.vi"("Tags to  Close"=w224, "Tree Refnum"=w228) -> ()  [unwired: 8 in, 2 out]
          }
          frame "Commands" {
            w237 = u32 5789784 ("Color Box")
            w238 = T27 {"Row"=-1, "Column"=-2} ("Active Cell:Active Cell")
            w240 = T27 {"Row"=-2, "Column"=-2} ("Active Cell:Active Cell")
            n122 = Index Array(array=w241, index=w235) -> (element=w239:u32)
            n123 = Index Array(array=w236, index=w235) -> (element=w234:T26)
            n124 = Unbundle(w234) -> ("Operation"=w233:enum16{"Update", "Clear"})  [unwired: 1 out]
            n125 = local read "Command Selection"() -> (w232:i32)
            n126 = property on="Command Selection" class="MCListbox (strict)"("ActiveCell"=w240, "CellBG"=w239, "ActiveCell"=w238, "CellBG"=w237) -> ()  [unwired: 2 in, 2 out]
            n127 = call <vilib>:"WPI_DashboardUpdate RPC Info.vi"("Operation"=w233) -> ("update"=w231:bool, "commands"=w230:string[][])  [unwired: 9 in]
            n128 = property on="Command Selection" class="MCListbox (strict)"("ItemNames"=w230) -> ()  [unwired: 2 in, 2 out]
            n129 = property on="Command Params" class="Tbl (strict)"("Active Cell"=w240, "Cell BG Color"=w239, "Active Cell"=w238, "Cell BG Color"=w237) -> ()  [unwired: 2 in, 2 out]
            n130 = call <vilib>:"WPI_DashboardUpdate Command Params.vi"("Update"=w231, "NewVal"=w232, "Commands"=w230, "Param Tbl"=w229) -> ()  [unwired: 7 in, 1 out]
          }
        }
        n131 = call <vilib>:"Connextion Info.vi"() -> ("Connected"=→"NT Connection":bool)  [unwired: 10 in, 1 out]
      }
      event "Test Tree": Value Change {
        # "Show appropriate\ncontrols"
        n132 = event-data() -> ("CtlRef"=w246:refnum<vi>, "NewVal"=w244:string)  [unwired: 1 in]
        n133 = call <vilib>:"WPI_UtilitiesGetTreeIOName.vi"("NewVal"=w244, "TreeControl in"=w246) -> ("I/O Name"=w247:string)  [unwired: 9 in]
        n134 = case shown="\"Camera\"" w247 {
          selector: w247 -> [_ w254 _ w276 w285 _]
          tunnel: w244 -> [_ _ w273 w275 _ w292]
          tunnel: cluster{string[]}[] [{["640x480", "320x240", "160x120"]}, {["Auto", "Fixed indoor", "Fixed outdoor 1", "Fixed outdoor 2", "Fixed fluorescent 1", "Fixed fluorescent 2", "Hold current"]}, {["Auto", "Flicker-free 50 Hz", "Flicker-free 60 Hz", "Hold current"]}, {["None", "Prioritize frame rate", "Prioritize image quality"]}, {["Monochrome", "Color"]}] -> [_ _ _ _ _ w291]
          frame Default {
            w249 = FALSE ("Visible")
            w248 = FALSE ("Visible")
            n135 = property on="Motor" class="Clust (strict)"("Visible"=w248) -> ()  [unwired: 2 in, 2 out]
            n136 = property on="Test Ring" class="Ring (strict)"("Visible"=w248) -> ()  [unwired: 2 in, 2 out]
            n137 = property on="Rev/Fwd" class="Clust (strict)"("Visible"=w249) -> ()  [unwired: 2 in, 2 out]
            n138 = property on="On/Off" class="Bool (strict)"("Visible"=w249) -> ()  [unwired: 2 in, 2 out]
            n139 = property on="Test Slider" class="Slide (strict)"("Visible"=w249) -> ()  [unwired: 2 in, 2 out]
          }
          frame "Analog Out", "Motor", "PWM" {
            w255 = FALSE ("Visible")
            n140 = case shown="\"Analog Out\"" w254 {
              tunnel: [1.0 ("Value") -1.0 ("Value") 0.0 ("Value")] -> w253
              tunnel: [255.0 ("Value") 1.0 ("Value") 5.0 ("Value")] -> w252
              tunnel: [128.0 ("Value") 0.0 ("Value") 0.0 ("Value")] -> w251
              tunnel: [64.0 ("Value") 0.5 ("Value") 1.0 ("Value")] -> w250
              frame "PWM" {
              }
              frame "Motor", Default {
              }
              frame "Analog Out" {
              }
            }
            n141 = property on="Motor" class="Clust (strict)"("Visible"=TRUE) -> ()  [unwired: 2 in, 2 out]
            n142 = property on="Value" class="Slide (strict)"("Value"=w251, "Scale.Minimum"=w253, "Scale.Maximum"=w252, "Scale.Increment"=w250) -> ()  [unwired: 2 in, 2 out]
            n143 = property on="On/Off" class="Bool (strict)"("Visible"=w255) -> ()  [unwired: 2 in, 2 out]
            n144 = property on="Test Slider" class="Slide (strict)"("Visible"=w255) -> ()  [unwired: 2 in, 2 out]
            n145 = property on="Test Ring" class="Ring (strict)"("Visible"=w255) -> ()  [unwired: 2 in, 2 out]
            n146 = property on="Rev/Fwd" class="Clust (strict)"("Visible"=w255) -> ()  [unwired: 2 in, 2 out]
          }
          frame "Servo" {
            w271 = FALSE ("Visible")
            n147 = call <vilib>:"NT Read Number.vi"("Name"=w273) -> ("Numeric"=w272:dbl)  [unwired: 9 in, 1 out]
            n148 = property on="Test Slider" class="Slide (strict)"("Visible"=TRUE, "Scale.Maximum"=170.0 ("Scale.Range:Maximum")) -> ()  [unwired: 2 in, 2 out]
            n149 = local write "Test Slider"(w272) -> ()
            n150 = property on="Motor" class="Clust (strict)"("Visible"=w271) -> ()  [unwired: 2 in, 2 out]
            n151 = property on="Rev/Fwd" class="Clust (strict)"("Visible"=w271) -> ()  [unwired: 2 in, 2 out]
            n152 = property on="On/Off" class="Bool (strict)"("Visible"=w271) -> ()  [unwired: 2 in, 2 out]
            n153 = property on="Test Ring" class="Ring (strict)"("Visible"=w271) -> ()  [unwired: 2 in, 2 out]
          }
          frame "Relay", "Solenoid" {
            w274 = FALSE ("Visible")
            n154 = property on="Motor" class="Clust (strict)"("Visible"=w274) -> ()  [unwired: 2 in, 2 out]
            n155 = property on="Test Slider" class="Slide (strict)"("Visible"=w274) -> ()  [unwired: 2 in, 2 out]
            n156 = Search and Replace String(input string=w275, search string="/Value  **", replace string="/Direction") -> (result string=w281:string)  [unwired: 5 in, 3 out]
            n157 = property on="Test Ring" class="Ring (strict)"("Visible"=w274) -> ()  [unwired: 2 in, 2 out]
            n158 = call <vilib>:"NT Read String.vi"("Name"=w281) -> ("String"=w279:string)  [unwired: 9 in, 1 out]
            n159 = Equal?(x="Both directions", y=w279) -> (x = y?=w277:bool)
            n160 = Not(x=w277) -> (.not. x?=w278:bool)
            n161 = property on="Rev/Fwd" class="Clust (strict)"("Visible"=w277) -> ()  [unwired: 2 in, 2 out]
            n162 = property on="On/Off" class="Bool (strict)"("Visible"=w278, "Caption.Text"=w276) -> ()  [unwired: 2 in, 2 out]
          }
          frame "Compressor", "Digital Out" {
            w284 = FALSE ("Visible")
            # "Get direction and finish"
            n163 = property on="Motor" class="Clust (strict)"("Visible"=w284) -> ()  [unwired: 2 in, 2 out]
            n164 = property on="Test Slider" class="Slide (strict)"("Visible"=w284) -> ()  [unwired: 2 in, 2 out]
            n165 = property on="Test Ring" class="Ring (strict)"("Visible"=w284) -> ()  [unwired: 2 in, 2 out]
            n166 = property on="On/Off" class="Bool (strict)"("Visible"=TRUE, "Caption.Text"=w285) -> ()  [unwired: 2 in, 2 out]
            n167 = property on="Rev/Fwd" class="Clust (strict)"("Visible"=FALSE) -> ()  [unwired: 2 in, 2 out]
          }
          frame "Camera" {
            n168 = call <vilib>:"Get Last Path Segment.vi"("String in"=w292) -> ("String out"=w293:string)  [unwired: 10 in]
            n169 = property on="On/Off" class="Bool (strict)"("Visible"=FALSE) -> ()  [unwired: 2 in, 2 out]
            n170 = property on="Motor" class="Clust (strict)"("Visible"=FALSE) -> ()  [unwired: 2 in, 2 out]
            n171 = property on="Rev/Fwd" class="Clust (strict)"("Visible"=FALSE) -> ()  [unwired: 2 in, 2 out]
            n172 = case shown="\"White Balance  **\"" w293 {
              tunnel: w292 -> [w299 w308 w317 w326 w335 _ w341]
              tunnel: w291 -> [w297 w305 w314 w323 w332 _ _]
              frame "Size  **" {
                n173 = Index Array(array=w297) -> (element=w296:cluster{string[]})  [unwired: 1 in]
                n174 = call <vilib>:"NT Read String.vi"("Name"=w299) -> ("String"=w298:string)  [unwired: 9 in, 1 out]
                n175 = Unbundle(w296) -> (w294:string[])
                n176 = Match First String(2:w294, 3:w298) -> (0:w295:i32)  [unwired: 1 out]
                n177 = property on="Test Ring" class="Ring (strict)"("Value"=w295, "Strings []"=w294) -> ()  [unwired: 2 in, 2 out]
                n178 = property on="Test Ring" class="Ring (strict)"("Visible"=TRUE) -> ()  [unwired: 2 in, 2 out]
                n179 = property on="Test Slider" class="Slide (strict)"("Visible"=FALSE) -> ()  [unwired: 2 in, 2 out]
              }
              frame "White Balance  **" {
                n180 = Index Array(array=w305, index=1) -> (element=w306:cluster{string[]})
                n181 = call <vilib>:"NT Read String.vi"("Name"=w308) -> ("String"=w307:string)  [unwired: 9 in, 1 out]
                n182 = Unbundle(w306) -> (w303:string[])
                n183 = Match First String(2:w303, 3:w307) -> (0:w302:i32)  [unwired: 1 out]
                n184 = property on="Test Ring" class="Ring (strict)"("Value"=w302, "Strings []"=w303) -> ()  [unwired: 2 in, 2 out]
                n185 = property on="Test Ring" class="Ring (strict)"("Visible"=TRUE) -> ()  [unwired: 2 in, 2 out]
                n186 = property on="Test Slider" class="Slide (strict)"("Visible"=FALSE) -> ()  [unwired: 2 in, 2 out]
              }
              frame "Exposure  **" {
                n187 = Index Array(array=w314, index=2) -> (element=w315:cluster{string[]})
                n188 = call <vilib>:"NT Read String.vi"("Name"=w317) -> ("String"=w316:string)  [unwired: 9 in, 1 out]
                n189 = Unbundle(w315) -> (w311:string[])
                n190 = Match First String(2:w311, 3:w316) -> (0:w312:i32)  [unwired: 1 out]
                n191 = property on="Test Ring" class="Ring (strict)"("Value"=w312, "Strings []"=w311) -> ()  [unwired: 2 in, 2 out]
                n192 = property on="Test Ring" class="Ring (strict)"("Visible"=TRUE) -> ()  [unwired: 2 in, 2 out]
                n193 = property on="Test Slider" class="Slide (strict)"("Visible"=FALSE) -> ()  [unwired: 2 in, 2 out]
              }
              frame "Exposure Priority  **" {
                n194 = Index Array(array=w323, index=3) -> (element=w324:cluster{string[]})
                n195 = call <vilib>:"NT Read String.vi"("Name"=w326) -> ("String"=w325:string)  [unwired: 9 in, 1 out]
                n196 = Unbundle(w324) -> (w320:string[])
                n197 = Match First String(2:w320, 3:w325) -> (0:w321:i32)  [unwired: 1 out]
                n198 = property on="Test Ring" class="Ring (strict)"("Value"=w321, "Strings []"=w320) -> ()  [unwired: 2 in, 2 out]
                n199 = property on="Test Ring" class="Ring (strict)"("Visible"=TRUE) -> ()  [unwired: 2 in, 2 out]
                n200 = property on="Test Slider" class="Slide (strict)"("Visible"=FALSE) -> ()  [unwired: 2 in, 2 out]
              }
              frame "Color Enable  **" {
                n201 = Index Array(array=w332, index=4) -> (element=w333:cluster{string[]})
                n202 = call <vilib>:"NT Read String.vi"("Name"=w335) -> ("String"=w334:string)  [unwired: 9 in, 1 out]
                n203 = Unbundle(w333) -> (w329:string[])
                n204 = Match First String(2:w329, 3:w334) -> (0:w330:i32)  [unwired: 1 out]
                n205 = property on="Test Ring" class="Ring (strict)"("Value"=w330, "Strings []"=w329) -> ()  [unwired: 2 in, 2 out]
                n206 = property on="Test Ring" class="Ring (strict)"("Visible"=TRUE) -> ()  [unwired: 2 in, 2 out]
                n207 = property on="Test Slider" class="Slide (strict)"("Visible"=FALSE) -> ()  [unwired: 2 in, 2 out]
              }
              frame Default {
                n208 = property on="Test Ring" class="Ring (strict)"("Visible"=FALSE) -> ()  [unwired: 2 in, 2 out]
                n209 = property on="Test Slider" class="Slide (strict)"("Visible"=FALSE) -> ()  [unwired: 2 in, 2 out]
              }
              frame "Brightness  **", "Color Level  **", "Compression  **", "FPS  **", "Sharpness  **" {
                n210 = call <vilib>:"NT Read Number.vi"("Name"=w341) -> ("Numeric"=w340:dbl)  [unwired: 9 in, 1 out]
                n211 = local write "Test Slider"(w340) -> ()
                n212 = property on="Test Slider" class="Slide (strict)"("Visible"=TRUE, "Scale.Maximum"=100.0 ("Scale.Range:Maximum")) -> ()  [unwired: 2 in, 2 out]
                n213 = property on="Test Ring" class="Ring (strict)"("Visible"=FALSE) -> ()  [unwired: 2 in, 2 out]
              }
            }
          }
        }
        n214 = property on="Progress" class="Clust (strict)"("Visible"=FALSE) -> ()  [unwired: 2 in, 2 out]
      }
      event "Test Name": Mouse Enter {
        # "Populate the ring with the list of tests"
        n215 = event-data() -> ()  [unwired: 1 in, 1 out]
        n216 = call <vilib>:"NT Read String Array.vi"("Name"="TestMode/TestList") -> ("String Array"=w349:string[])  [unwired: 9 in, 1 out]
        n217 = Build Array (concatenate)("Select the test to run...", w349) -> (w348:string[])
        n218 = property on="Test Name" class="Ring (strict)"("Strings []"=w348) -> ()  [unwired: 2 in, 2 out]
      }
      event "Test Name": Value Change {
        w351 = FALSE ("Visible")
        # "Tell the robot the test name to run"
        n219 = event-data() -> ("NewVal"=w355:u16)  [unwired: 1 in]
        n220 = property on="Test Name" class="Ring (strict)"() -> ("Strings []"=w356:string[])  [unwired: 2 in, 2 out]
        n221 = local write "Progress"(T6 {"Test Progress"=0, "Test Progress Text"=""} ("Progress")) -> ()
        n222 = Index Array(array=w356, index=w355) -> (element=w354:string)
        n223 = call <vilib>:"NT Write String.vi"("String"=w354, "Name"="TestMode/TestName") -> ()  [unwired: 9 in, 1 out]
        n224 = property on="Progress" class="Clust (strict)"("Visible"=TRUE) -> ()  [unwired: 2 in, 2 out]
        n225 = property on="Motor" class="Clust (strict)"("Visible"=w351) -> ()  [unwired: 2 in, 2 out]
        n226 = property on="Test Slider" class="Slide (strict)"("Visible"=w351) -> ()  [unwired: 2 in, 2 out]
        n227 = property on="On/Off" class="Bool (strict)"("Visible"=w351) -> ()  [unwired: 2 in, 2 out]
        n228 = property on="Rev/Fwd" class="Clust (strict)"("Visible"=w351) -> ()  [unwired: 2 in, 2 out]
        n229 = property on="Test Ring" class="Ring (strict)"("Visible"=w351) -> ()  [unwired: 2 in, 2 out]
      }
      event "Select Auto": Mouse Enter {
        # "Populate the combo box with the list of autonomous options"
        n230 = event-data() -> ()  [unwired: 1 in, 1 out]
        n231 = call <vilib>:"NT Read String Array.vi"("Name"="Auto List") -> ("String Array"=w358:string[])  [unwired: 9 in, 1 out]
        n232 = property on="Select Auto" class="CmbBox"("Strings[]"=w358) -> ()  [unwired: 2 in, 2 out]
      }
      event "Select Auto": Value Change {
        # "User modified the Auto Selection. Write to NT variable so robot knows."
        n233 = event-data() -> ("NewVal"=w361:string)  [unwired: 1 in]
        n234 = call <vilib>:"NT Write String.vi"("String"=w361, "Name"="Auto Selector") -> ()  [unwired: 9 in, 1 out]
      }
      event "Command Selection": Value Change {
        # "Get the params and show in table"
        n235 = event-data() -> ("NewVal"=w367:i32)  [unwired: 1 in]
        n236 = property on="Command Selection" class="MCListbox (strict)"() -> ("ItemNames"=w365:string[][])  [unwired: 2 in, 2 out]
        n237 = call <vilib>:"WPI_DashboardUpdate Command Params.vi"("NewVal"=w367, "Commands"=w365, "Param Tbl"=w366) -> ()  [unwired: 8 in, 1 out]
      }
      event "Execute Command": Value Change {
        # "Started one, Unique ID holds\nresponse"
        n238 = event-data() -> ()  [unwired: 1 in, 1 out]
        n239 = property on="Command Selection" class="MCListbox (strict)"() -> ("ItemNames"=w378:string[][])  [unwired: 2 in, 2 out]
        n240 = Index Array(array=w378, index (row)="Command Selection", index (col)=0) -> (element=w376:string)
        n241 = call <vilib>:"Invoke Commands.vi"("Command Params"="Command Params", "Function Name"=w376) -> ("Params"=w372:u8, "Started"=w371:bool)  [unwired: 7 in, 1 out]
        n242 = Array Subset(array="Command Params", length (row)=w372) -> (w373:string[][])  [unwired: 3 in]
        n243 = Select(t="Executing" ("Cmd Status"), s=w371, f="" ("Cmd Status")) -> (s? t:f=→"Cmd Status":string)
      }
      event "Command Selection": Double Click {
        n244 = event-data() -> ("Row"=w386:i32)  [unwired: 1 in]
        n245 = property on="Command Selection" class="MCListbox (strict)"() -> ("ItemNames"=w389:string[][])  [unwired: 2 in, 2 out]
        n246 = local read "Command Params"() -> (w385:string[][])
        n247 = Index Array(array=w389, index (row)=w386, index (col)=0) -> (element=w387:string)
        n248 = call <vilib>:"Invoke Commands.vi"("Command Params"=w385, "Function Name"=w387) -> ("Params"=w384:u8, "Started"=w379:bool)  [unwired: 7 in, 1 out]
        n249 = Array Subset(array=w385, length (row)=w384) -> (w383:string[][])  [unwired: 3 in]
        n250 = Select(t="Executing" ("Cmd Status"), s=w379, f="" ("Cmd Status")) -> (s? t:f=w380:string)
        n251 = local write "Cmd Status"(w380) -> ()
      }
      event "CheckList": Double Click {
        # "Shift clears all"
        # "Update symbols on the listbox"
        n252 = event-data() -> ("PlatMods.Shift"=w391:bool, "Row"=w393:i32)  [unwired: 1 in]
        n253 = case shown="True" w391 {
          tunnel: w393 -> [w397 _]
          tunnel: 1 -> [w396 _]
          frame False {
            n254 = property on="CheckList" class="LstBox (strict)"() -> ("Item Symbols"=w395:i32[])  [unwired: 2 in, 2 out]
            n255 = Replace Array Subset(array=w395, new element=w396, index=w397) -> (w394:i32[])
            n256 = property on="CheckList" class="LstBox (strict)"("Item Symbols"=w394) -> ()  [unwired: 2 in, 2 out]
          }
          frame True {
            w398 = 0 ("Top Row")
            n257 = property on="CheckList" class="LstBox (strict)"() -> ("Number of Rows"=w400:u32)  [unwired: 2 in, 2 out]
            n258 = Initialize Array(0, w400) -> (w399:i32[])
            n259 = property on="CheckList" class="LstBox (strict)"("Top Row"=w398, "Value"=w398, "Item Symbols"=w399) -> ()  [unwired: 2 in, 2 out]
          }
        }
      }
      event "CheckList": Key Down {
        # "Update symbols on the listbox\nLeft and right keys check and uncheck"
        n260 = event-data() -> ("VKey"=w404:T24)  [unwired: 1 in]
        n261 = case shown="\"Left\", \"Right\"" w404 {
          selector: w404 -> [w409 _]
          tunnel: eventvkey."Left" ("VKey") -> [w407 _]
          frame "Left", "Right" {
            n262 = Equal?(x=w407, y=w409) -> (x = y?=w408:bool)
            n263 = Select(t=0, s=w408, f=1) -> (s? t:f=w410:i32)
            n264 = property on="CheckList" class="LstBox (strict)"() -> ("Item Symbols"=w413:i32[])  [unwired: 2 in, 2 out]
            n265 = Replace Array Subset(array=w413, new element=w410, index="CheckList") -> (w412:i32[])
            n266 = property on="CheckList" class="LstBox (strict)"("Item Symbols"=w412) -> ()  [unwired: 2 in, 2 out]
          }
          frame Default {
          }
        }
      }
      event "Motor.Enable": Value Change {
        # "When the test mode otor enable helper is set, update that\ntree row item's value"
        n267 = event-data() -> ("NewVal"=w419:bool)  [unwired: 1 in]
        n268 = Unbundle("Motor") -> ("Value"=w418:dbl)  [unwired: 1 out]
        n269 = Select(t=w418, s=w419, f=0.0) -> (s? t:f=w416:dbl)
        n270 = call <vilib>:"NT Write Number.vi"("Numeric"=w416, "Name"=w415) -> ()  [unwired: 9 in, 1 out]
      }
      event "Test Slider": Value Change {
        # "When the test mode slider helper is set, update that\ntree row item's value"
        n271 = event-data() -> ("NewVal"=w422:dbl)  [unwired: 1 in]
        n272 = call <vilib>:"NT Write Number.vi"("Numeric"=w422, "Name"=w423) -> ()  [unwired: 9 in, 1 out]
      }
      event "On/Off": Value Change {
        # "When the test mode on/off helper value is set, update that\ntree row item's value"
        n273 = event-data() -> ("NewVal"=w427:bool)  [unwired: 1 in]
        n274 = Boolean To (0,1)(Boolean=w427) -> (0, 1=w426:i16)
        n275 = call <vilib>:"NT Write Number.vi"("Numeric"=w426, "Name"=w425) -> ()  [unwired: 9 in, 1 out]
      }
      event "Rev/Fwd": Value Change {
        # "When the test mode helper value for relays is set, update that\ntree row item's value"
        n276 = event-data() -> ("NewVal.Forward"=w435:bool, "NewVal.Reverse"=w434:bool)  [unwired: 1 in]
        n277 = Boolean To (0,1)(Boolean=w435) -> (0, 1=w431:i16)
        n278 = Boolean To (0,1)(Boolean=w434) -> (0, 1=w433:i16)
        n279 = Negate(x=w433) -> (-x=w432:i16)
        n280 = Add(x=w431, y=w432) -> (x+y=w430:i16)
        n281 = call <vilib>:"NT Write Number.vi"("Numeric"=w430, "Name"=w429) -> ()  [unwired: 9 in, 1 out]
      }
      event "Test Ring": Value Change {
        # "When a test mode helper value is selected from the ring,\nset the tree item's variable to the string value"
        n282 = event-data() -> ("NewVal"=w439:u16)  [unwired: 1 in]
        n283 = property on="Test Ring" class="Ring (strict)"() -> ("Strings []"=w440:string[])  [unwired: 2 in, 2 out]
        n284 = Index Array(array=w440, index=w439) -> (element=w438:string)
        n285 = call <vilib>:"NT Write String.vi"("String"=w438, "Name"=w437) -> ()  [unwired: 9 in, 1 out]
      }
      event "Rec Mode": Value Change {
        # "Update globals for recording mode and path to read log from.\nClear when logging and let NetworkTables set path for vision to\nuse."
        n286 = event-data() -> ("NewVal"=w451:enum32{"Stop", "Record", "Playback"})  [unwired: 1 in]
        n287 = global write "WPI_DashboardLogging Global.vi" "Logging Filename"(path "") -> ()
        n288 = global write "WPI_DashboardLogging Global.vi" "Recording"(w451) -> ()
        n289 = case shown="\"Playback\"" w451 {
          tunnel: w450 -> [_ w453 w462]
          tunnel: [_ _ w461] -> w448
          tunnel: [_ _ w460] -> _
          tunnel: w446 -> [_ _ w458]
          tunnel: cluster{i32, i32} {-250, 170} -> [_ _ w457]
          tunnel: [_ _ T25 {"Image Size"=TRUE, "Image Type"=TRUE, "Pixel Value"=TRUE, "ROI Information"=TRUE, "Zoom Factor"=FALSE} ("Image Information Shown:All Elements")] -> w441
          tunnel: [_ _ TRUE ("Zoom Factor")] -> w442
          tunnel: w444 -> [_ _ w454]
          frame Default {
          }
          frame "Stop", "Record" {
            # "Place Window too"
            n290 = invoke class="VI" method="FP.Close"(reference=w453) -> (reference out=w452:refnum<vi>)  [unwired: 2 in, 2 out]
            n291 = invoke class="VI" method="Abort VI"(reference=w452) -> ()  [unwired: 2 in, 3 out]
          }
          frame "Playback" {
            n292 = call "Open Playback Panel.vi"("Offset"=w457, "DB VI Ref"=w458, "Playback in"=w462) -> ("Playback out"=w459:refnum<vi>)  [unwired: 8 in]
            n293 = register-events(w459, w454) -> (reference out=w461:refnum<event-registration>, error out=w460:errorcluster)  [unwired: 2 in]
          }
        }
        n294 = property on="Camera Image Right" class="ImageControl"("Image Information Shown"=w441, "Image Information Visible"=w442) -> ()  [unwired: 2 in, 2 out]
        n295 = property on="Camera Image" class="ImageControl"("Image Information Shown"=w441, "Image Information Visible"=w442) -> ()  [unwired: 2 in, 2 out]
        n296 = call <vilib>:"WPI_DashboardNT Log FieldName Cache.vi"("Operation"=enum16{"Lookup/Add", "Index", "Clear"}."Clear") -> ()  [unwired: 8 in, 3 out]
      }
      event Panel Close {
        w464 = enum32{"Stop", "Record", "Playback"}."Stop" ("Rec Mode")
        # "Playback window has been closed, abort"
        n297 = event-data() -> ()  [unwired: 1 in, 4 out]
        n298 = local write "Rec Mode"(w464) -> ()
        n299 = global write "WPI_DashboardLogging Global.vi" "Recording"(w464) -> ()
      }
      event Panel Close {
        # "Abort playback window and ourself"
        n300 = event-data() -> ()  [unwired: 1 in, 4 out]
        n301 = invoke class="VI" method="FP.Close"(reference=w468) -> (reference out=w467:refnum<vi>)  [unwired: 2 in, 2 out]
        n302 = invoke class="VI" method="Abort VI"(reference=w467) -> (error out=w466:errorcluster)  [unwired: 2 in, 2 out]
        n303 = invoke class="VI" method="Abort VI"(error in=w466) -> ()  [unwired: 2 in, 3 out]
      }
      event User Event {
        n304 = event-data() -> ("IDs"=w475:cluster{"RPC field ID":u16, "Unique ID":u16}, "String"=w474:string)  [unwired: 1 in]
        n305 = Bundle("IDs"=w475, "String"=w474) -> (w473:T9)  [unwired: 1 in]
        n306 = call <vilib>:"Retrieve RPC Response.vi"("RPC Response"=w473) -> ("Output"=w471:string[][])  [unwired: 10 in]
        n307 = Build Array (concatenate)(w469, w471) -> (w470:string[][])
        n308 = local write "Command Params"(w470) -> ()
        n309 = local write "Cmd Status"("" ("Cmd Status")) -> ()
      }
      event "Tree": Double Click {
        n310 = event-data() -> ("PlatMods"=w481:T28, "Tag"=w478:string)  [unwired: 1 in]
        n311 = Unbundle(w481) -> ("Shift"=w480:bool)  [unwired: 4 out]
        n312 = String Subset(string=w478, length (rest)=1 ("length (rest)")) -> (substring=w477:string)  [unwired: 1 in]
        n313 = Not(x=w480) -> (.not. x?=w479:bool)
        n314 = case shown="\"/\"" w477 {
          tunnel: w478 -> [_ w484]
          tunnel: w479 -> [_ w483]
          frame Default {
          }
          frame "/" {
            n315 = call <vilib>:"NT Update Persistence.vi"("Persistence"=w483, "Name"=w484) -> ()  [unwired: 9 in, 1 out]
          }
        }
      }
    }
  }
  n316 = while {
    tunnel: w65 -> [w486]
    i -> [w489]
    stop <- FALSE stop-if-true
    n317 = Wait (ms)(milliseconds to wait=u32 100) -> ()  [unwired: 1 out]
    n318 = case shown="\"Playback\"" "Rec Mode" {
      tunnel: w489 -> [_ _ w504]
      tunnel: [u32 2829099 ("Base Color") u32 11141120 ("Target Color") w493] -> w485
      frame "Stop", Default {
        # "Reset the color, extra updates don't cost much"
      }
      frame "Record" {
      }
      frame "Playback" {
        # "Playback"
        n319 = Quotient & Remainder(x=w504, y=u32 50 ("milliseconds to wait")) -> (x-y*floor(x/y)=w500:u32)  [unwired: 1 out]
        n320 = Divide(x=w500, y=u32 50 ("milliseconds to wait")) -> (x/y=w497:dbl)
        n321 = Multiply(x=6.283185307179586, y=w497) -> (x*y=w502:dbl)
        n322 = Sine(x=w502) -> (sin(x)=w501:dbl)
        n323 = Absolute Value(x=w501) -> (abs(x)=w494:dbl)
        n324 = call "Interpolate RGB Color.vi"("Proportion"=w494, "Target Color"=u32 30976, "Base Color"=u32 2829099) -> ("Result Color"=w493:u32)  [unwired: 8 in]
      }
    }
    n325 = property class="Pane"(reference=w486, "PaneColor"=w485) -> ()  [unwired: 1 in, 2 out]
  }
  n326 = local write "Dashboard Tab"(T2."Drive" ("Dashboard Tab")) -> ()
  n327 = property on="On/Off" class="Bool (strict)"("Visible"=w36) -> ()  [unwired: 2 in, 2 out]
  n328 = property on="Motor" class="Clust (strict)"("Visible"=w36) -> ()  [unwired: 2 in, 2 out]
  n329 = property on="Progress" class="Clust (strict)"("Visible"=w36) -> ()  [unwired: 2 in, 2 out]
  n330 = property on="Test Ring" class="Ring (strict)"("Visible"=w36) -> ()  [unwired: 2 in, 2 out]
  n331 = property on="Rev/Fwd" class="Clust (strict)"("Visible"=w36) -> ()  [unwired: 2 in, 2 out]
  n332 = while {
    tunnel: u16 1741 ("timeout ms (25000)") -> [w506]
    stop <- FALSE stop-if-true
    n333 = TCP Create Listener(10:w506) -> (0:w505:errorcluster, 3:w507:refnum<k5>)  [unwired: 4 in, 1 out]
    n334 = case shown="No Error" w505 {
      selector: w505 -> [w509 _]
      tunnel: w507 -> [w510 _]
      frame No Error {
        n335 = while {
          tunnel: w510 -> [w513]
          tunnel: w509 -> [w512]
          stop <- FALSE stop-if-true
          n336 = TCP Wait On Listener(8:w512, 11:w513) -> (0:w514:errorcluster, 4:w515:refnum<k5>)  [unwired: 2 in, 3 out]
          n337 = local write "TCP"(w515) -> ()
          n338 = case shown="No Error" w514 {
            frame No Error {
            }
            frame Error {
              n339 = Wait (ms)(milliseconds to wait=u32 1000) -> ()  [unwired: 1 out]
            }
          }
        }
      }
      frame Error {
        n340 = Wait (ms)(milliseconds to wait=u32 1000) -> ()  [unwired: 1 out]
      }
    }
  }
  n341 = local write "Command Selection"(u16 0 ("milliseconds to wait")) -> ()
  n342 = local write "Command Params"(string[][] [] ("Command Params")) -> ()
  n343 = global write "WPI_DashboardLogging Global.vi" "Recording"(w59) -> ()
  n344 = local write "Rec Mode"(w59) -> ()
  n345 = call <vilib>:"NT Write String.vi"("String"="Select Auto", "Name"="Auto Selector") -> ()  [unwired: 9 in, 1 out]
